vi "Global Data Id Prefix.vi"() -> ()   [LabVIEW 2023, in "RFCalAndFixtureCharact.Common.lvlib"]
uses:
  RFCalAndFixtureCharact.Common.lvlib
panel:
  in  "InstrumentModels":string="InstrumentModels"
  in  "VNAInstrumentTypeId":string="RFINST_VNA"
  in  "RFPMPresent":string="RFPMPresent"
  in  "ColdSourceDUT":string="ColdSourceDUT"
  in  "FPGAVIReferences":string="FPGAVIReferences"
  in  "ResourceDescriptors":string="ResourceDescriptors"
  in  "RefClkSource":string="RefClkSource"
  in  "RFDCData":string="RFDCData_"
  in  "SequenceDirectory":string="SequenceDirectory_"
  in  "WaveformAttributes":string="WaveformAttributes_"
  in  "WaveformName":string="WaveformName_"
  in  "SAMode":string="SAMode_"
  in  "EnableDeembedding":string="EnableDeembedding_"
  in  "SGMode":string="SGMode_"
  in  "FirstDUTStatus":string="FirstDUTStatus_"
  in  "ServoResult":string="ServoResult_"
  in  "rfsts_":string="rfsts_"
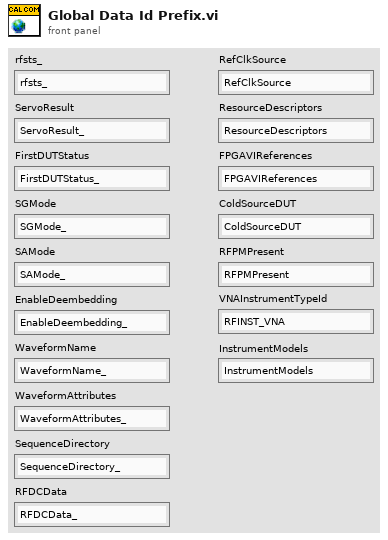
[diagram p1: front panel]
diagram:
